vi "Init Coil Calibration.vi"(5 "Magnet ID":string, 6 "# Power Supplies":u32(slide)=4 min=1 max=4 step=1 scale=1.0..4.0) -> (0 "Magnet Configuration Data":T1 {"Scale Factors" format="%.3f"; "Offsets" format="%.3f"; "Temp Coef" format="%.4g"; "Maximum Coil Currents" format="%.2g"; "Coil Inductances" format="%.3g"; "Pressure Range" format="%.2f"}, 1 "P Scale Max":dbl, 2 "P Scale Min":dbl, 3 "I Scale Max":dbl, 4 "File Name":string)   [LabVIEW 2020]
doc: "Reads configuration file for the selected magnet from the folder \"Magnet Calibrations\" on the system disk. All comments (lines starting with a '#') are stripped out and the configuration parameters are parsed and output.\nScott Hannahs, NHMFL-FSU, April 1995"
uses:
  Sub Controls/RMPS Magnet Config.ctl
  RMPS Globals.vi
panel:
  # "Tin"
  # "Tout"
  # "Pin"
  # "Pout"
  # "I"
  # "WDTin"
  # "PSEnb"
  # "CellFLT"
  # "WDTout"
  # "BTFlt"
  # "BTvolt"
  # "Va"
  # "Vb"
  # "Vc"
  # "Vd"
  # "Tin"
  # "Tout"
  # "Pin"
  # "Pout"
  # "I"
  # "WDTin"
  # "PSEnb"
  # "CellFLT"
  # "WDTout"
  # "BTFlt"
  # "BTvolt"
  # "Va"
  # "Vb"
  # "Vc"
  # "Vd"
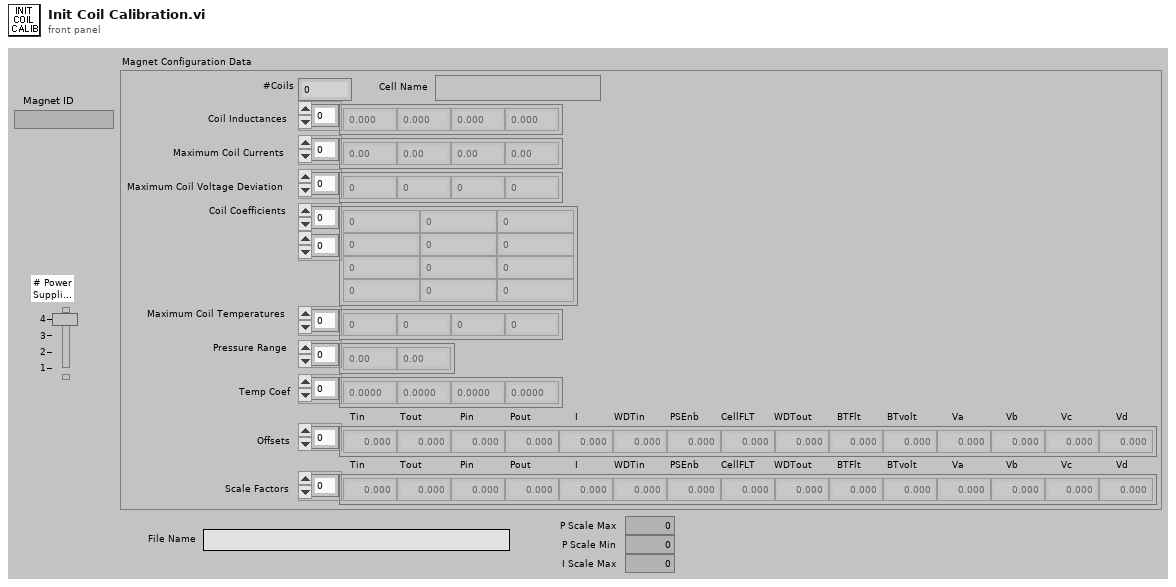
[diagram p1: front panel]
types:
  T1 = typedef "RMPS Magnet Config.ctl" = cluster{"#Coils":u32, "Coil Inductances":dbl[], "Maximum Coil Currents":dbl[], "Maximum Coil Voltage Deviation":dbl[], "Coil Coefficients":dbl[][], "Maximum Coil Temperatures":dbl[], " Pressure Range":dbl[], "Temp Coef":dbl[], "Offsets":dbl[], "Scale Factors":dbl[], "Cell Name":string}
  T2 = cluster{u32, sgl[], sgl[], sgl[], sgl[][], sgl[], sgl[], sgl[], sgl[], sgl[], "Magnet ID":string}
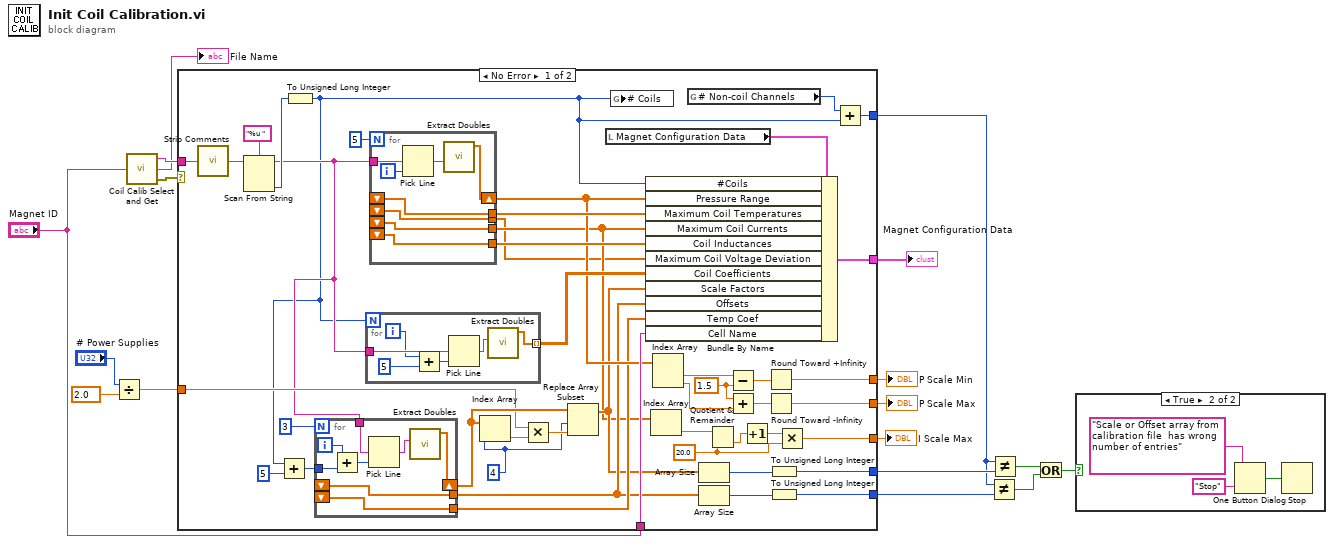
[diagram p0: block diagram]
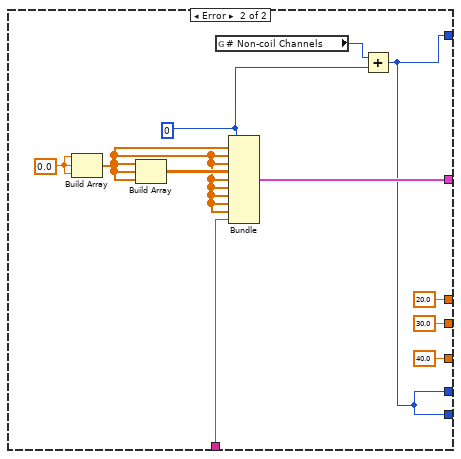
[diagram p3: hidden frame]
diagram:
  n1 = Divide(x="# Power Supplies", y=sgl 2.0) -> (x/y=w13:sgl)
  n2 = call "Coil Calib Select and Get.vi"("Magnet ID"="Magnet ID") -> ("String"=w12:string, "File Name"=→"File Name":string, "error out"=w11:errorcluster)
  n3 = case shown="No Error" w11 {
    tunnel: "Magnet ID" -> [w47 w95]
    tunnel: [w45 w92] -> w17
    tunnel: w12 -> [w54 _]
    tunnel: w13 -> [w55 _]
    tunnel: [w37 20.0] -> w10
    tunnel: [w36 30.0] -> w9
    tunnel: [w28 w85] -> w7
    tunnel: [w29 w85] -> w8
    tunnel: [w31 w85] -> w6
    tunnel: [w20 40.0] -> w2
    frame No Error {
      w21 = 20.0 ("y")
      w40 = 1.5 ("y")
      w25 = u32 4 ("y")
      n4 = call "Strip Comments.vi"(1:w54) -> (0:w50:string)
      n5 = Scan From String(format string="%u ", input string=w50) -> (remaining string=w51:string, output 1=w52:u32)  [unwired: 3 in, 2 out]
      n6 = To Unsigned Long Integer(number=w52) -> (unsigned 32bit integer=w32:u32)
      n7 = Add(x=w32, y=u32 5) -> (x+y=w59:u32)
      n8 = for {
        N: 3 -> [_]
        shift-right: [w66] -> w56
        shift-left: _ -> [w68]
        shift-left: _ -> [w67]
        tunnel: [w68] -> w35
        tunnel: [w67] -> w27
        tunnel: w51 -> [w69]
        tunnel: w59 -> [w63]
        i -> [w64]
        n9 = Add(x=w64, y=w63) -> (x+y=w65:u32)
        n10 = Pick Line(multi-line string=w69, line index=w65) -> (output string=w70:string)  [unwired: 1 in]
        n11 = call "Extract Doubles.vi"("String"=w70) -> ("Data"=w66:dbl[])  [unwired: 5 in, 1 out]
      }
      n12 = for {
        N: w32 -> [_]
        tunnel: w51 -> [w75]
        tunnel: [w74] -> w44 mode=indexing
        i -> [w72]
        n13 = Add(x=w72, y=5) -> (x+y=w73:i32)
        n14 = Pick Line(multi-line string=w75, line index=w73) -> (output string=w76:string)  [unwired: 1 in]
        n15 = call "Extract Doubles.vi"("String"=w76) -> ("Data"=w74:dbl[])  [unwired: 5 in, 1 out]
      }
      n16 = for {
        N: 5 -> [_]
        shift-right: [w77] -> w43
        shift-left: _ -> [w79]
        shift-left: _ -> [w81]
        shift-left: _ -> [w80]
        shift-left: _ -> [w78]
        tunnel: [w79] -> w46
        tunnel: [w81] -> w24
        tunnel: [w80] -> w18
        tunnel: [w78] -> w48
        tunnel: w51 -> [w83]
        i -> [w82]
        n17 = Pick Line(multi-line string=w83, line index=w82) -> (output string=w84:string)  [unwired: 1 in]
        n18 = call "Extract Doubles.vi"("String"=w84) -> ("Data"=w77:dbl[])  [unwired: 5 in, 1 out]
      }
      n19 = Index Array(array=w56, index=w25) -> (element=w58:dbl)
      n20 = Multiply(x=w55, y=w58) -> (x*y=w57:dbl)
      n21 = Replace Array Subset(array=w56, new element=w57, index=w25) -> (w26:dbl[])
      n22 = local read "Magnet Configuration Data"() -> (w49:T1)
      n23 = global write "RMPS Globals.vi" "# Coils"(w32) -> ()
      n24 = Bundle By Name(cluster=w49, "#Coils"=w32, "Pressure Range"=w43, "Maximum Coil Temperatures"=w48, "Maximum Coil Currents"=w24, "Coil Inductances"=w46, "Maximum Coil Voltage Deviation"=w18, "Coil Coefficients"=w44, "Scale Factors"=w26, "Offsets"=w27, "Temp Coef"=w35, "Cell Name"=w47) -> (w45:T1)
      n25 = Index Array(array=w24) -> (element=w23:dbl)  [unwired: 1 in]
      n26 = Index Array(array=w43) -> (element #1=w42:dbl, element #2=w41:dbl)  [unwired: 2 in]
      n27 = global read "RMPS Globals.vi" "# Non-coil Channels"() -> (w30:u32)
      n28 = Array Size(array=w26) -> (size(s)=w33:i32)
      n29 = Array Size(array=w27) -> (size(s)=w34:i32)
      n30 = Quotient & Remainder(x=w23, y=w21) -> (floor(x/y)=w22:dbl)  [unwired: 1 out]
      n31 = Subtract(x=w42, y=w40) -> (x-y=w39:dbl)
      n32 = Add(x=w40, y=w41) -> (x+y=w38:dbl)
      n33 = Increment(x=w22) -> (x+1=w19:dbl)
      n34 = Round Toward +Infinity(x=w39) -> (ceil(x): smallest int >= x=w37:dbl)
      n35 = Round Toward -Infinity(1:w38) -> (0:w36:dbl)
      n36 = To Unsigned Long Integer(number=w33) -> (unsigned 32bit integer=w29:u32)
      n37 = To Unsigned Long Integer(number=w34) -> (unsigned 32bit integer=w28:u32)
      n38 = Multiply(x=w19, y=w21) -> (x*y=w20:dbl)
      n39 = Add(x=w30, y=w32) -> (x+y=w31:u32)
    }
    frame Error {
      w87 = u32 0
      w94 = sgl 0.0
      n40 = Build Array(w94, w94, w94) -> (w89:sgl[])
      n41 = Build Array(w89, w89, w89) -> (w93:sgl[][])
      n42 = global read "RMPS Globals.vi" "# Non-coil Channels"() -> (w88:u32)
      n43 = Bundle(w87, w89, w89, w89, w93, w89, w89, w89, w89, w89, "Magnet ID"=w95) -> (w92:T2)  [unwired: 1 in]
      n44 = Add(x=w88, y=w87) -> (x+y=w85:u32)
    }
  }
  "Magnet Configuration Data" <- w17
  "P Scale Min" <- w10
  "P Scale Max" <- w9
  "I Scale Max" <- w2
  n45 = Not Equal?(x=w6, y=w7) -> (x != y?=w4:bool)
  n46 = Not Equal?(x=w6, y=w8) -> (x != y?=w5:bool)
  n47 = Or(x=w5, y=w4) -> (x .or. y?=w3:bool)
  n48 = case shown="True" w3 {
    frame False {
    }
    frame True {
      n49 = One Button Dialog(message="Scale or Offset array from calibration file  has wrong number of entries", button name ("OK")="Stop") -> (true=w98:bool)
      n50 = Stop(stop? (T)=w98) -> ()
    }
  }
